vi "indicatorVisibility4Ch.vi"(7 "device type [AB1004]":T2=1004 items=["any"=0, "AB1002"=1002, "AB1004"=1004, "AB1502"=1502, "AB1504"=1504, "AB2002"=2002, "AB2004"=2004, "AB2502"=2502, "AB2504"=2504], 9 "ref indics":T1, 10 "connection state":T3) -> ()   [LabVIEW 2015]
doc: "Sets the visibility of indicators on front panel at \"Tausand AB1000 Acquisition Example.vi\", depending on the current connection state."
uses:
  <instrlib>/Tausand AB1000/Examples/sub vi/connectionState.ctl
  <instrlib>/Tausand AB1000/Public/Controls/deviceTypeRing.ctl
  <instrlib>/Tausand AB1000/Tausand AB1000.lvlib
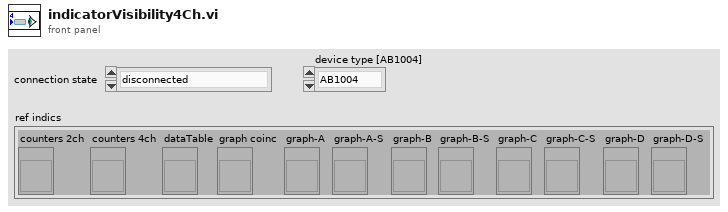
[diagram p1: front panel]
types:
  T1 = cluster{"counters 2ch":refnum<vi>, "counters 4ch":refnum<vi>, "dataTable":refnum<vi>, "graph coinc":refnum<vi>, "graph-A":refnum<vi>, "graph-A-S":refnum<vi>, "graph-B":refnum<vi>, "graph-B-S":refnum<vi>, "graph-C":refnum<vi>, "graph-C-S":refnum<vi>, "graph-D":refnum<vi>, "graph-D-S":refnum<vi>}
  T2 = typedef "Tausand AB1000.lvlib/deviceTypeRing.ctl" = u16
  T3 = typedef "connectionState.ctl" = enum16{"disconnected", "connected", "acquiring data", "connection error", "acquisition error"}
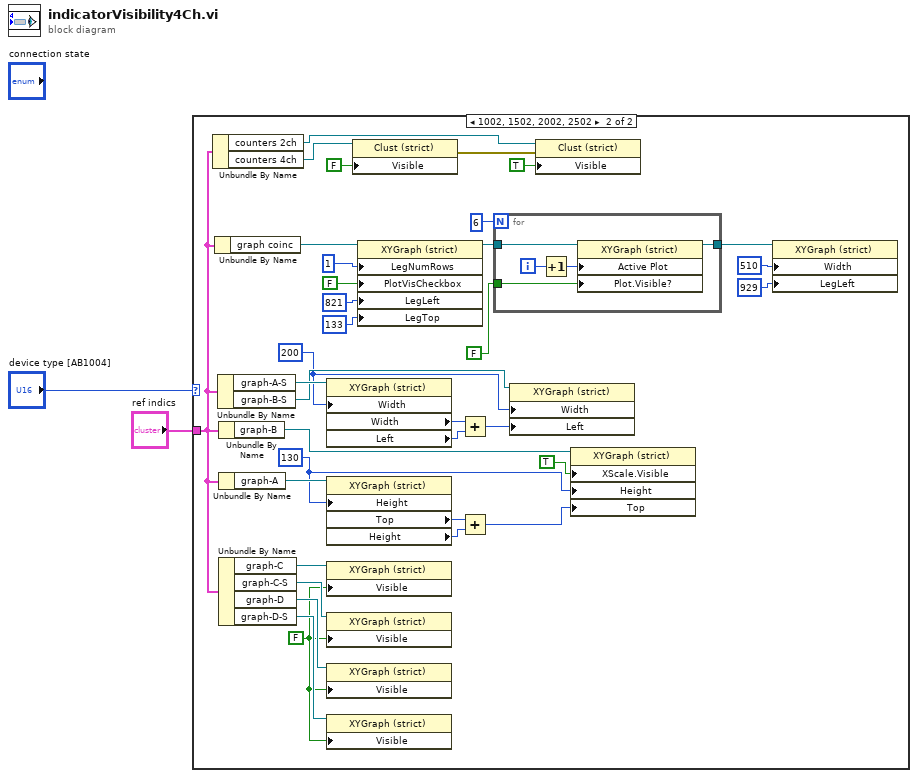
[diagram p0: block diagram]
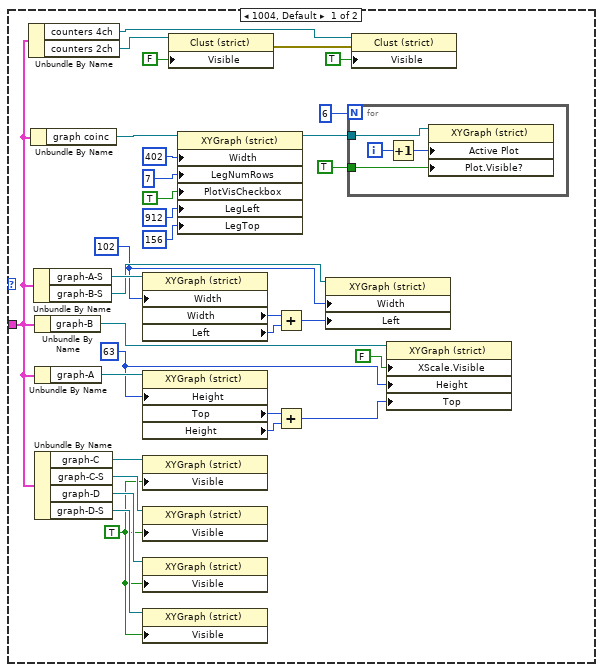
[diagram p2: hidden frame]
diagram:
  n1 = case shown="1002, 1502, 2002, 2502" "device type [AB1004]" {
    tunnel: "ref indics" -> [w6 w55]
    frame 1004, Default {
      w4 = u32 102 ("Plot Area:Size:Width")
      w21 = u32 63 ("Plot Area:Size:Height")
      w28 = TRUE ("Visible")
      n2 = Unbundle By Name(w6) -> ("counters 4ch"=w26:refnum<vi>, "counters 2ch"=w27:refnum<vi>)
      n3 = Unbundle By Name(w6) -> ("graph coinc"=w16:refnum<vi>)
      n4 = Unbundle By Name(w6) -> ("graph-A-S"=w10:refnum<vi>, "graph-B-S"=w9:refnum<vi>)
      n5 = Unbundle By Name(w6) -> ("graph-B"=w25:refnum<vi>)
      n6 = Unbundle By Name(w6) -> ("graph-A"=w23:refnum<vi>)
      n7 = Unbundle By Name(w6) -> ("graph-C"=w32:refnum<vi>, "graph-C-S"=w31:refnum<vi>, "graph-D"=w30:refnum<vi>, "graph-D-S"=w29:refnum<vi>)
      n8 = property class="XYGraph (strict)"(reference=w10, "Width"=w4) -> ("Width"=w8:u32, "Left"=w7:i32)  [unwired: 1 in, 2 out]
      n9 = property class="XYGraph (strict)"(reference=w23, "Height"=w21) -> ("Top"=w22:i32, "Height"=w19:u32)  [unwired: 1 in, 2 out]
      n10 = property class="XYGraph (strict)"(reference=w32, "Visible"=w28) -> ()  [unwired: 1 in, 2 out]
      n11 = property class="XYGraph (strict)"(reference=w31, "Visible"=w28) -> ()  [unwired: 1 in, 2 out]
      n12 = property class="XYGraph (strict)"(reference=w30, "Visible"=w28) -> ()  [unwired: 1 in, 2 out]
      n13 = property class="XYGraph (strict)"(reference=w29, "Visible"=w28) -> ()  [unwired: 1 in, 2 out]
      n14 = property class="Clust (strict)"(reference=w27, "Visible"=FALSE) -> (error out=w34:errorcluster)  [unwired: 1 in, 1 out]
      n15 = property class="XYGraph (strict)"(reference=w16, "Width"=u32 402 ("Plot Area:Size:Width"), "LegNumRows"=u32 7 ("Legend:Number of Rows"), "PlotVisCheckbox"=TRUE ("Legend:Plot Visibility Checkbox Visible"), "LegLeft"=912 ("Legend:Position:Left"), "LegTop"=156 ("Legend:Position:Top")) -> (reference out=w3:refnum<vi>)  [unwired: 1 in, 1 out]
      n16 = Add(x=w8, y=w7) -> (x+y=w5:u32)
      n17 = Add(x=w22, y=w19) -> (x+y=w20:u32)
      n18 = property class="XYGraph (strict)"(reference=w9, "Width"=w4, "Left"=w5) -> ()  [unwired: 1 in, 2 out]
      n19 = for {
        N: 6 -> [_]
        tunnel: w3 -> [w39]
        tunnel: TRUE ("X Scale.Visible") -> [w36]
        i -> [w38]
        n20 = Increment(x=w38) -> (x+1=w37:i32)
        n21 = property class="XYGraph (strict)"(reference=w39, "Active Plot"=w37, "Plot.Visible?"=w36) -> ()  [unwired: 1 in, 2 out]
      }
      n22 = property class="Clust (strict)"(reference=w26, error in=w34, "Visible"=TRUE) -> ()  [unwired: 2 out]
      n23 = property class="XYGraph (strict)"(reference=w25, "XScale.Visible"=FALSE ("X Scale.Visible"), "Height"=w21, "Top"=w20) -> ()  [unwired: 1 in, 2 out]
    }
    frame 1002, 1502, 2002, 2502 {
      w52 = u32 200 ("Plot Area:Size:Width")
      w60 = u32 130 ("Plot Area:Size:Height")
      w67 = FALSE ("Visible")
      n24 = Unbundle By Name(w55) -> ("counters 2ch"=w65:refnum<vi>, "counters 4ch"=w66:refnum<vi>)
      n25 = Unbundle By Name(w55) -> ("graph coinc"=w47:refnum<vi>)
      n26 = Unbundle By Name(w55) -> ("graph-A-S"=w54:refnum<vi>, "graph-B-S"=w53:refnum<vi>)
      n27 = Unbundle By Name(w55) -> ("graph-B"=w64:refnum<vi>)
      n28 = Unbundle By Name(w55) -> ("graph-A"=w62:refnum<vi>)
      n29 = Unbundle By Name(w55) -> ("graph-C"=w71:refnum<vi>, "graph-C-S"=w70:refnum<vi>, "graph-D"=w69:refnum<vi>, "graph-D-S"=w68:refnum<vi>)
      n30 = property class="XYGraph (strict)"(reference=w54, "Width"=w52) -> ("Width"=w51:u32, "Left"=w50:i32)  [unwired: 1 in, 2 out]
      n31 = property class="XYGraph (strict)"(reference=w62, "Height"=w60) -> ("Top"=w61:i32, "Height"=w58:u32)  [unwired: 1 in, 2 out]
      n32 = property class="XYGraph (strict)"(reference=w71, "Visible"=w67) -> ()  [unwired: 1 in, 2 out]
      n33 = property class="XYGraph (strict)"(reference=w70, "Visible"=w67) -> ()  [unwired: 1 in, 2 out]
      n34 = property class="XYGraph (strict)"(reference=w69, "Visible"=w67) -> ()  [unwired: 1 in, 2 out]
      n35 = property class="XYGraph (strict)"(reference=w68, "Visible"=w67) -> ()  [unwired: 1 in, 2 out]
      n36 = property class="Clust (strict)"(reference=w66, "Visible"=FALSE) -> (error out=w73:errorcluster)  [unwired: 1 in, 1 out]
      n37 = property class="XYGraph (strict)"(reference=w47, "LegNumRows"=u32 1 ("Legend:Number of Rows"), "PlotVisCheckbox"=FALSE ("Legend:Plot Visibility Checkbox Visible"), "LegLeft"=821 ("Legend:Position:Left"), "LegTop"=133 ("Legend:Position:Top")) -> (reference out=w46:refnum<vi>)  [unwired: 1 in, 1 out]
      n38 = Add(x=w51, y=w50) -> (x+y=w49:u32)
      n39 = Add(x=w61, y=w58) -> (x+y=w59:u32)
      n40 = for {
        N: 6 -> [_]
        tunnel: w46 -> [w79]
        tunnel: FALSE ("X Scale.Visible") -> [w76]
        tunnel: [w75] -> w43
        i -> [w78]
        n41 = Increment(x=w78) -> (x+1=w77:i32)
        n42 = property class="XYGraph (strict)"(reference=w79, "Active Plot"=w77, "Plot.Visible?"=w76) -> (reference out=w75:refnum<vi>)  [unwired: 1 in, 1 out]
      }
      n43 = property class="XYGraph (strict)"(reference=w53, "Width"=w52, "Left"=w49) -> ()  [unwired: 1 in, 2 out]
      n44 = property class="Clust (strict)"(reference=w65, error in=w73, "Visible"=TRUE) -> ()  [unwired: 2 out]
      n45 = property class="XYGraph (strict)"(reference=w64, "XScale.Visible"=TRUE ("X Scale.Visible"), "Height"=w60, "Top"=w59) -> ()  [unwired: 1 in, 2 out]
      n46 = property class="XYGraph (strict)"(reference=w43, "Width"=u32 510 ("Plot Area:Size:Width"), "LegLeft"=929 ("Legend:Position:Left")) -> ()  [unwired: 1 in, 2 out]
    }
  }
